vi "QX_StartDaq.vi"(0 "DaqMeasurement":refnum<k24>, 7 "SyncTimeout":i32=2000, 9 "AcquisitionMode":i32, 11 "Error in":errorcluster) -> (4 "DaqMeasurement":refnum<k24>, 8 "MaxTimeDelta":dbl, 15 "Error out":errorcluster)   [LabVIEW 2016]
doc: "Starts (synchronized) measurement of all signals that were added to the measurement. \n\n\nDevicesAndSignal: Devices and Signals that are used for the measurement (just passed through).\nMaxTimeDelta: Maximum difference between time stamps of the first measurement values. 0 means, that the first time stamp of each signal has the same value.\nSyncTimeout: Maximum time in ms, that is used to start a synchronized measurement. If it is not possible to start a synchronized measurement within this time, an error will be thrown. \nAcquisitionMode: Modus of the data acquisition. \nSoftwareSynchronized = 0\nHardwareSynchronized = 1\nUnsynchronized = 2\nUse SoftwareSynchronized, if first timestamp of all signals should be as close as possible to each other. Therefore the devices have to be synchronized! Use HardwareSynchrnonized, if the devices are synchronized by hardware (cable) and deliver a common first timestamp for each signal. Use Unsynchronized to start a measurement without a common first timestamp for all signals (in that case syncTimeOut is not taken into account and the function returns with 0.0)"
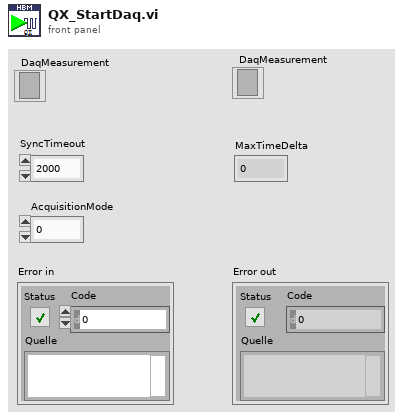
[diagram p1: front panel]
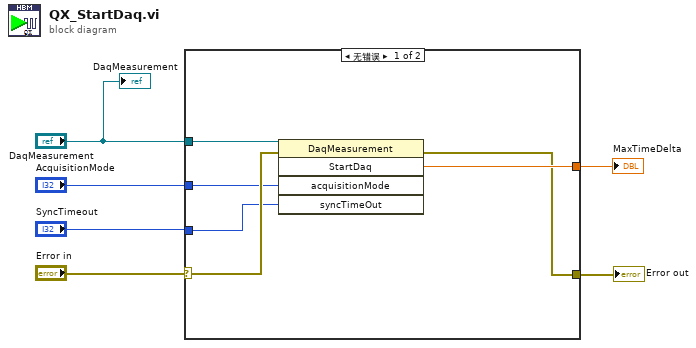
[diagram p0: block diagram]
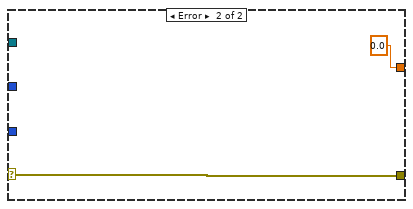
[diagram p2: hidden frame]
diagram:
  n1 = case shown="无错误" "Error in" {
    selector: "Error in" -> [w12 w14]
    tunnel: "DaqMeasurement" -> [w7 _]
    tunnel: [w8 w14] -> w5
    tunnel: "SyncTimeout" -> [w11 _]
    tunnel: "AcquisitionMode" -> [w10 _]
    tunnel: [w9 0.0 ("StartDaq")] -> w2
    frame No Error {
      n2 = invoke on="Methodenknoten" class="DaqMeasurement" method="StartDaq"(reference=w7, error in=w12, "acquisitionMode"=w10, "syncTimeOut"=w11) -> (error out=w8:errorcluster, "StartDaq"=w9:dbl)  [unwired: 1 in, 3 out]
    }
    frame Error {
    }
  }
  "Error out" <- w5
  "MaxTimeDelta" <- w2
  "DaqMeasurement" <- "DaqMeasurement"
